vi "Stitching-Output image setup window.vi"(6 "Min":cluster{"X min (um) ":dbl, "Y min (um)":dbl}, 9 "Canvas Y size in":i32, 11 "Canvas X size in":i32) -> (0 "Cancelled?":bool, 3 "Size reduction multiplier":dbl)   [LabVIEW 2013]
doc: "Use this template to create a dialog box with event handling."
uses:
  Global Variables/General Globals.vi
panel:
  in  "Output resolution":dbl(slide) step=0.01 scale=0.01..1.0
  in  "Cancel":bool
  out "Output Y size":i32 format="Output image Y: %.0f pixels"
  out "Output X size":i32 format="Output image X: %.0f pixels"
  in  "OK":bool
  # "Output Images Setup"
  # "Max (original)"
  # "Min"
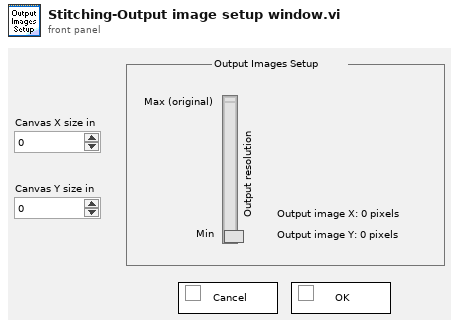
[diagram p1: front panel]
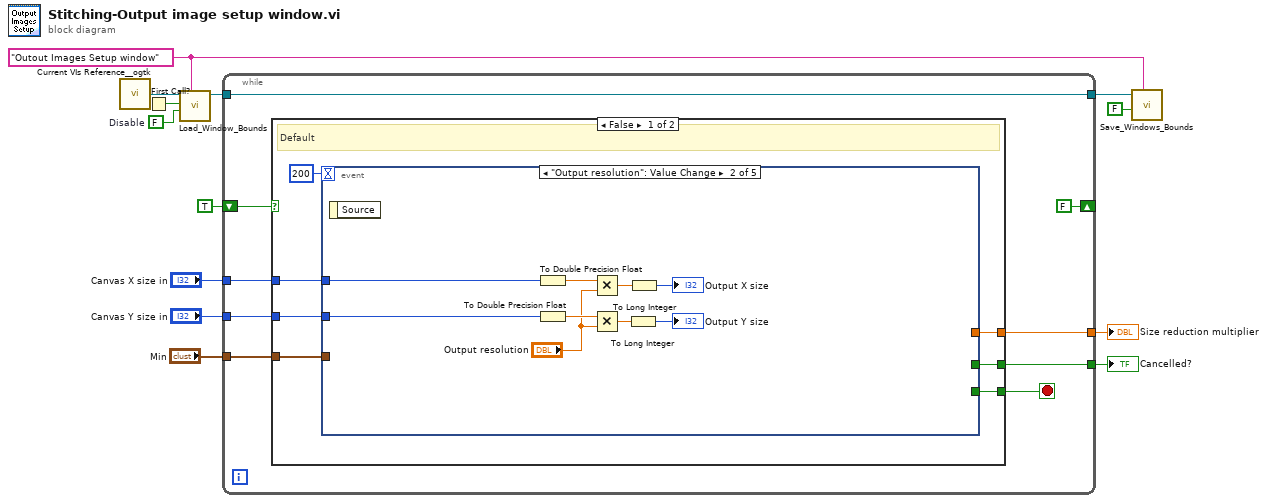
[diagram p0: block diagram]
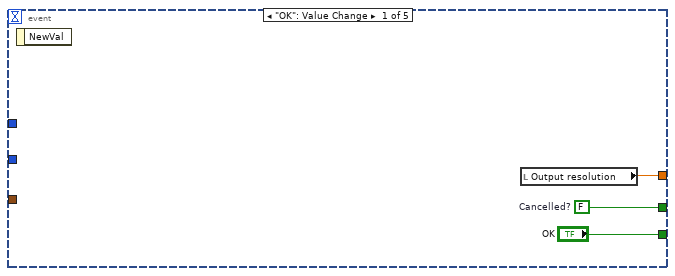
[diagram p2: hidden frame]
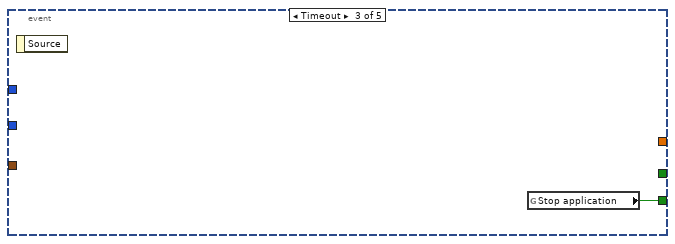
[diagram p3: hidden frame]
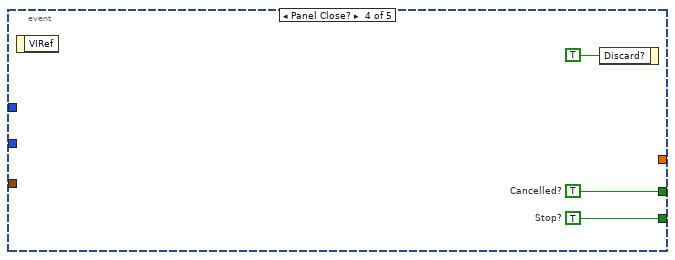
[diagram p4: hidden frame]
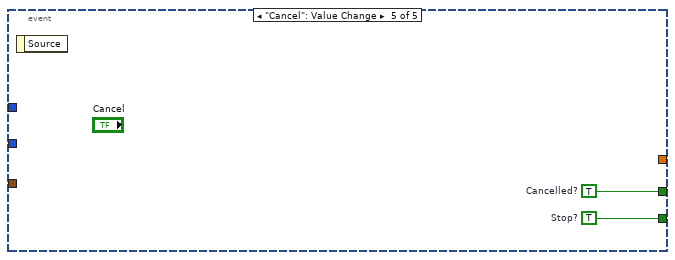
[diagram p5: hidden frame]
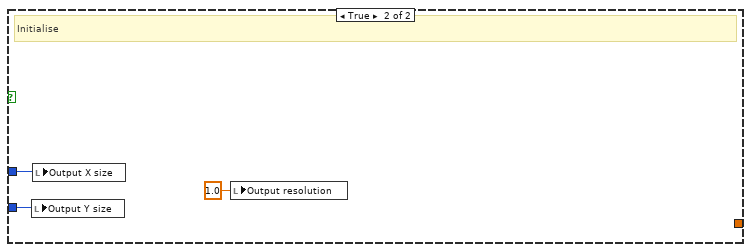
[diagram p6: hidden frame]
diagram:
  w9 = FALSE  # Disable
  w8 = "Outout Images Setup window" ("Window Name (i.e. Key)")
  n1 = call "Current VIs Reference__ogtk.vi"() -> ("Current VI's reference"=w11:refnum<vi>)  [unwired: 5 in]
  n2 = First Call?() -> (First Call?: T/F=w10:bool)
  n3 = call "Load_Window_Bounds.vi"("Window Name (i.e. Key)"=w8, "Disable"=w9, "First Call"=w10, "Window VI's Ref"=w11) -> ("reference out"=w6:refnum<vi>)  [unwired: 4 in, 3 out]
  n4 = while {
    tunnel: [w21] -> w13
    shift-right: [FALSE] -> _
    shift-left: TRUE -> [w20]
    tunnel: w6 -> [w18]
    tunnel: [w18] -> w5
    tunnel: "Canvas Y size in" -> [w17]
    tunnel: "Canvas X size in" -> [w16]
    tunnel: "Min" -> [w15]
    tunnel: [w14] -> w1
    stop <- w22 stop-if-true
    n5 = case shown="False" w20 {
      tunnel: [w29 _] -> w22
      tunnel: [w28 _] -> w21
      tunnel: w17 -> [w26 w49]
      tunnel: w16 -> [w25 w50]
      tunnel: w15 -> [w24 _]
      tunnel: [w23 _] -> w14
      frame False {
        # "Default"
        n6 = event shown="[1] \"Output resolution\": Value Change" {
          selector: _ -> [_ _ _ _ _]
          dyn-events: _ -> [_ _ _ _ _]
          timeout: 200 -> [_ _ _ _ _]
          tunnel: ["OK" _ w42 w44 w47] -> w29
          tunnel: [w32 _ _ w43 w46] -> w28
          tunnel: w26 -> [_ w38 _ _ _]
          tunnel: w25 -> [_ w41 _ _ _]
          tunnel: w24 -> [_ _ _ _ _]
          tunnel: [w30 _ _ _ _] -> w23
          event "OK": Value Change {
            w32 = FALSE  # Cancelled?
            n7 = event-data() -> ()  [unwired: 1 in, 1 out]
            n8 = local read "Output resolution"() -> (w30:dbl)
          }
          event "Output resolution": Value Change {
            n9 = event-data() -> ()  [unwired: 1 in, 1 out]
            n10 = To Double Precision Float(number=w41) -> (double precision float=w40:dbl)
            n11 = To Double Precision Float(number=w38) -> (double precision float=w39:dbl)
            n12 = Multiply(x=w40, y="Output resolution") -> (x*y=w37:dbl)
            n13 = Multiply(x=w39, y="Output resolution") -> (x*y=w36:dbl)
            n14 = To Long Integer(number=w36) -> (32bit integer=→"Output Y size":i32)
            n15 = To Long Integer(number=w37) -> (32bit integer=→"Output X size":i32)
          }
          event Timeout {
            n16 = event-data() -> ()  [unwired: 1 in, 1 out]
            n17 = global read "General Globals.vi" "Stop application"() -> (w42:bool)
          }
          event Panel Close? {
            w43 = TRUE  # Cancelled?
            w44 = TRUE  # Stop?
            n18 = event-data() -> ()  [unwired: 1 in, 1 out]
            n19 = event-data("Discard?"=TRUE) -> ()  [unwired: 1 in, 1 out]
          }
          event "Cancel": Value Change {
            w46 = TRUE  # Cancelled?
            w47 = TRUE  # Stop?
            n20 = event-data() -> ()  [unwired: 1 in, 1 out]
          }
        }
      }
      frame True {
        # "Initialise"
        n21 = local write "Output Y size"(w49) -> ()
        n22 = local write "Output X size"(w50) -> ()
        n23 = local write "Output resolution"(1.0 ("Output resolution")) -> ()
      }
    }
  }
  "Cancelled?" <- w13
  "Size reduction multiplier" <- w1
  n24 = call "Save_Windows_Bounds.vi"("Window Name (i.e. Key)"=w8, "Front Panel Window:Open"=FALSE, "Window VI's Ref"=w5) -> ()  [unwired: 8 in, 1 out]
